vi "Get Open Weather Session DVR.vi"(8 "Error In":errorcluster, 11 "Open Weather Session In":refnum<class "Open Weather Session.lvclass">) -> (0 "Error Out":errorcluster, 2 "DVR":refnum<data-value>, 3 "Open Weather Session Out":refnum<class "Open Weather Session.lvclass">)   [LabVIEW 2019, in "Open Weather Session.lvclass"]
uses:
  Open Weather Session.lvclass
  Controls/Data.ctl
  <vilib>/addons/_JKI.lib/REST Client/classes/REST Client/REST Client.lvclass
  Open Weather Session.lvclass/Open Weather Session.ctl
  Utilities/Open Weather Utilities.lvlib
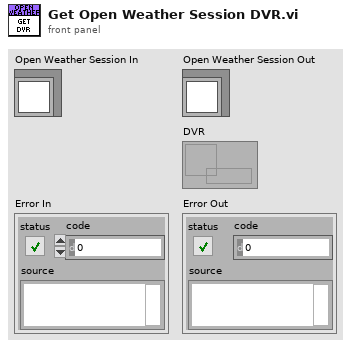
[diagram p1: front panel]
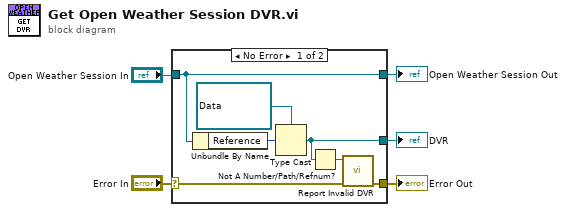
[diagram p0: block diagram]
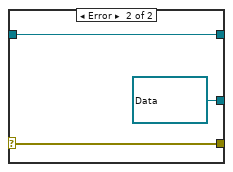
[diagram p2: hidden frame]
diagram:
  n1 = case shown="No Error" "Error In" {
    selector: "Error In" -> [w8 w15]
    tunnel: "Open Weather Session In" -> [w11 w14]
    tunnel: [w7 w15] -> w3
    tunnel: [w11 w14] -> w2
    tunnel: [w6 refnum<data-value> refnum ("data value reference")] -> w1
    frame No Error {
      n2 = Unbundle By Name(w11) -> ("Reference"=w12:u64)
      n3 = Type Cast(type=refnum<data-value> refnum ("data value reference"), x=w12) -> (*(type *) &x=w6:refnum<data-value>)
      n4 = Not A Number/Path/Refnum?(number/path/refnum=w6) -> (NaN/Path/Refnum?=w9:bool)
      n5 = call "Report Invalid DVR.vi"("Error In"=w8, "Invalid DVR"=w9) -> ("Error Out"=w7:errorcluster)  [unwired: 9 in]
    }
    frame Error {
    }
  }
  "Error Out" <- w3
  "Open Weather Session Out" <- w2
  "DVR" <- w1
